vi "Cursor Unset Busy.vi"(8 "error in (no error)":errorcluster, 11 "LF2R IDE in":refnum<class "LF2R IDE.lvclass">) -> (0 "error out":errorcluster, 3 "LF2R IDE out":refnum<class "LF2R IDE.lvclass">)   [LabVIEW 2018, in "LF2R IDE.lvlib" / "LF2R IDE.lvclass"]
uses:
  LF2R IDE.lvclass
  LF2R IDE.lvclass/LF2R IDE.ctl
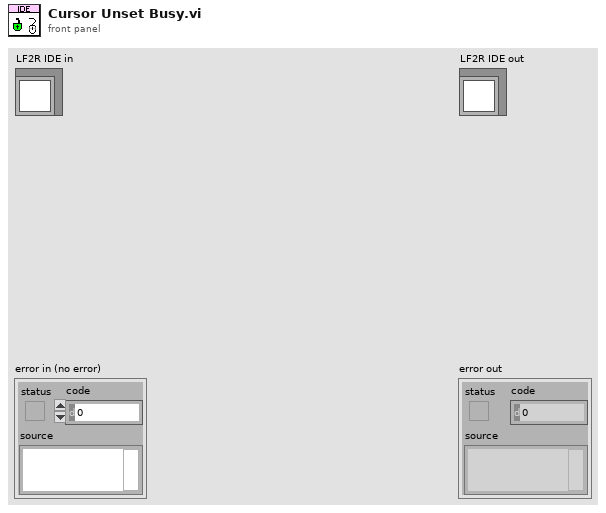
[diagram p1: front panel]
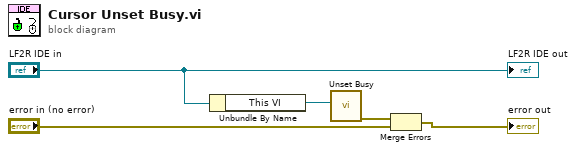
[diagram p0: block diagram]
diagram:
  n1 = Unbundle By Name("LF2R IDE in") -> ("This VI"=w2:refnum<vi>)
  n2 = call <vilib>:"Unset Busy.vi"("VI reference (current VI)"=w2) -> ("error out"=w1:errorcluster)  [unwired: 10 in]
  n3 = Merge Errors(w1, "error in (no error)") -> (→"error out":errorcluster)
  "LF2R IDE out" <- "LF2R IDE in"
